vi "niScope Probe Compensation Signal Start.vi"(0 "instrument handle":refnum<k15>, 11 "error in":errorcluster) -> (4 "instrument handle out":refnum<k15>, 15 "error out":errorcluster)   [LabVIEW 2011]
doc: "Starts the 1 kHz square wave output on PFI 1 for probe compensation."
uses:
  niScope_32.dll
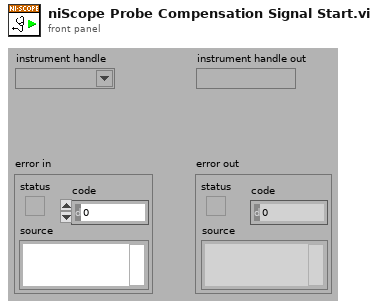
[diagram p1: front panel]
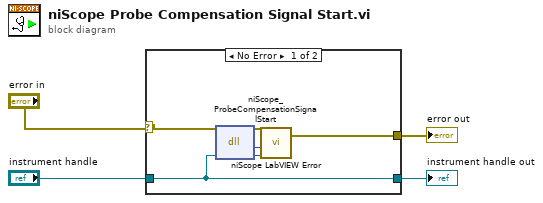
[diagram p0: block diagram]
diagram:
  n1 = case shown="No Error" "error in" {
    selector: "error in" -> [w5 w10]
    tunnel: [w7 w10] -> w4
    tunnel: [w6 w11] -> w2
    tunnel: "instrument handle" -> [w6 w11]
    frame No Error {
      n2 = dll-call lib="niScope_*.*" fn="niScope_ProbeCompensationSignalStart"("instrument handle"=w6) -> ("status"=w8:i32, "instrument handle"=w9:u32)  [unwired: 3 in, 2 out]
      n3 = call <instrlib>:"niScope LabVIEW Error.vi"("instrument handle"=w9, "niScope error code (0)"=w8, "error in (no error)"=w5) -> ("error out"=w7:errorcluster)  [unwired: 2 in]
    }
    frame Error {
    }
  }
  "error out" <- w4
  "instrument handle out" <- w2
